vi "TCP Read.vi"(7 "Timeout (1000 ms )":i32=1000, 8 "Error In":errorcluster, 10 "Bytes To Read":i32=4, 11 "LINX Device Config":T1={"Interface"=enum."TCP", "COM Port"="COM5", "TCP Configuration"={"IP Address"="10.2.106.213", "Port"=6921}, "Device Family"=1, "Device ID"=1, "Device Name"="chipKIT uC32", "TCP Ref"=refnum, "Channels"={"DI"=[], "DO"=[], "AI"=[], "AO"=[], "PWM"=[], "QE"=[], "UART"=[], "I2C 2"=[], "SPI"=[], "CAN"=[], "Servo"=[], "AI Ref (V)"=0.0, "AO Ref (V)"=0.0, "AO Resolution (Bits)"=0}}) -> (0 "Error Out":errorcluster, 2 "Data":string, 3 "LINX Device Config":T1={"Interface"=enum."TCP", "COM Port"="COM5", "TCP Configuration"={"IP Address"="10.2.106.213", "Port"=6921}, "Device Family"=1, "Device ID"=1, "Device Name"="chipKIT uC32", "TCP Ref"=refnum, "Channels"={"DI"=[], "DO"=[], "AI"=[], "AO"=[], "PWM"=[], "QE"=[], "UART"=[], "I2C 2"=[], "SPI"=[], "CAN"=[], "Servo"=[], "AI Ref (V)"=0.0, "AO Ref (V)"=0.0, "AO Resolution (Bits)"=0}})   [LabVIEW 2011, in "LMH-LINX.lvlib" / "Device.lvlib"]
uses:
  Device.lvlib
  Type Defs/LINX Device Config.ctl
  Type Defs/Interface.ctl
  Type Defs/TCP Config.ctl
  Type Defs/Channels.ctl
  LMH-LINX.lvlib
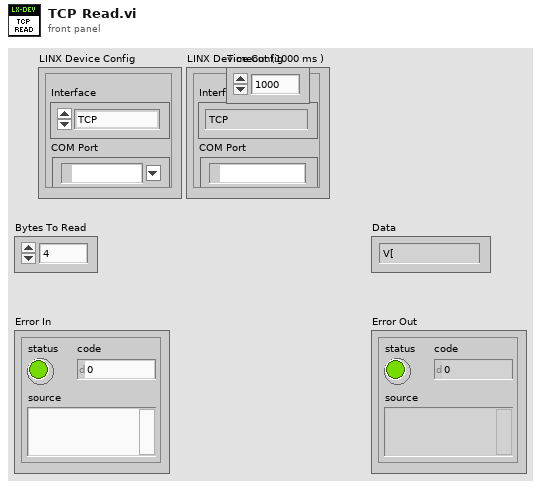
[diagram p1: front panel]
types:
  T1 = typedef "LMH-LINX.lvlib/Device.lvlib/LINX Device Config.ctl" = cluster{"Interface":T2, "COM Port":refnum<visa-resource-name>, "TCP Configuration":T3, "Device Family":u8, "Device ID":u8, "Device Name":string, "TCP Ref":refnum<k5>, "Channels":T4}
  T2 = typedef "LMH-LINX.lvlib/Interface.ctl" = enum16{"Serial", "TCP"}
  T3 = typedef "LMH-LINX.lvlib/Device.lvlib/TCP Config.ctl" = cluster{"IP Address":string, "Port":u16}
  T4 = typedef "LMH-LINX.lvlib/Channels.ctl" = cluster{"DI":u8[], "DO":u8[], "AI":u8[], "AO":u8[], "PWM":u8[], "QE":u8[], "UART":u8[], "I2C 2":u8[], "SPI":u8[], "CAN":u8[], "Servo":u8[], "AI Ref (V)":dbl, "AO Ref (V)":dbl, "AO Resolution (Bits)":u8}
  T5 = enum16{"Standard", "Buffered", "CRLF", "Immediate"}
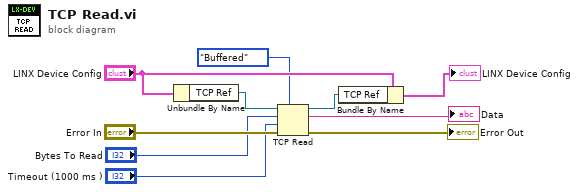
[diagram p0: block diagram]
diagram:
  n1 = Unbundle By Name("LINX Device Config") -> ("TCP Ref"=w5:refnum<k5>)
  n2 = TCP Read(connection ID=w5, bytes to read="Bytes To Read", error in (no error)="Error In", 7:T5."Buffered" ("mode (standard)"), 9:"Timeout (1000 ms )") -> (connection ID out=w8:refnum<k5>, data out=→"Data":string, error out=→"Error Out":errorcluster)
  n3 = Bundle By Name(cluster="LINX Device Config", "TCP Ref"=w8) -> (→"LINX Device Config":T1)
